vi "IO Test.vi"() -> ()   [LabVIEW 2009]
doc: "This example shows how to use Simulation Module and Control Design Toolkit together and how to transfer the controller from Design to Simulation. It also uses the 3D Picture Control Toolkit to animate the system.\nThis example is derived from the Quanser (www.quanser.com) 3 DOF Helicopter academic experiment."
uses:
  <vilib>/Simulation/Scripting/Companion Diagram/SimConfigNode/SimDog.xnode
  <vilib>/Simulation/Utility/SIMX Halt/SIMX Halt.xnode
  <vilib>/Simulation/Implementation/Shared/SIMSCR Execution Mode.ctl
  <vilib>/Simulation/Scripting/Companion Diagram/SimConfigNode/_simSolvers.ctl
  <vilib>/Simulation/Scripting/Companion Diagram/SimConfigNode/SimParams.ctl
  <vilib>/Simulation/Utility/Implementation/SIM Halt.vi
  NiRioSrv.dll
  <vilib>/Utility/error.llb/Error Cluster From Error Code.vi
  <vilib>/rvi/errors/niLvFpgaWhatHappensToTopLevelVI.ctl
  <vilib>/rvi/interface/common/niFpgaNodeNameForErrorReporting.ctl
  <vilib>/rvi/errors/niLvFpgaAdjustHostInterfaceError.vi
  <vilib>/rvi/interface/nirviReadWriteControl/nirviReadWriteControl.xnode
  FPGA Bitfiles/sbRIOController.lv~4B_sbRIO-9631_FPGA Main.vi.lvbitx
  <vilib>/userDefined/High Color/nirio_resource_hc.ctl
  <vilib>/rvi/interface/nirviOpenFPGA/nirviOpenFPGA.xnode
  RT/Set to PWM.vi
  <vilib>/rvi/interface/nirviCloseFPGA/nirviCloseFPGA.xnode
  FPGA/FPGA Main.vi
  RT/Read Encoder Data.vi
  <vilib>/Simulation/Implementation/Shared/SIM Bundle Sim Info.vi
  <vilib>/Simulation/Implementation/Shared/SIM Unbundle Sim Info.vi
  <vilib>/Platform/TimedLoop/XDataNode/wakeup.ctl
  <vilib>/Platform/TimedLoop/XDataNode/XDNodeRunTimeDep.lvlib
  <vilib>/Platform/TimedLoop/XDataNode/nitl_modes.ctl
  <vilib>/Platform/TimedLoop/XDataNode/timing_clust.ctl
  <vilib>/Platform/TimedLoop/XDataNode/XDataNode.xnode
  <vilib>/Simulation/Implementation/Shared/NILVSim_Initialize.vi
  <vilib>/Simulation/Implementation/Shared/NILVSim_FinishedLate.vi
  <vilib>/Simulation/Implementation/Shared/NILVSim_Manager.vi
  <vilib>/Simulation/Implementation/Shared/NILVSim_FinalizeModel.vi
  <vilib>/Simulation/Implementation/Shared/NILVSim_GetModelError.vi
  <vilib>/Platform/TimedLoop/XDataNode/loadlvalarms.vi
  <vilib>/Simulation/Implementation/Shared/SIM Fire Discrete SubVI.vi
  <vilib>/Simulation/Scripting/Editor Utilities/SIM subVI execution type.ctl
  <vilib>/Simulation/Scripting/Editor Utilities/SIM subVI tag data.ctl
  <vilib>/FPGAPlugInAG/sbRIO-9631/nirviIntfOpen_sbRIO-9631.vi
  FPGA/FPGA Main NoStartEnc.vi
  FPGA Bitfiles/sbRIOController.lv~4B_sbRIO-9631_FPGA Main NoStartE~C3.lvbitx
  <vilib>/FPGAPlugInAG/sbRIO-9631/nirviIntfClose_sbRIO-9631.vi
panel:
  in  "Fan Power (-1 to 1) 2":dbl(slide) scale=-1.0..1.0
  out "Trav Vel":dbl
  out "Pitch Vel":dbl
  out "Elv Vel":dbl
  in  "Fan Power (-1 to 1)":dbl(slide) scale=-1.0..1.0
  in  "stop":bool
  out "error out":errorcluster
  in  "GO":bool
  in  "Clock Divider (ticks)":u16=1
  in  "PWM Period (ticks)":u32=100000
  out "Measured Pitch Angle":dbl=0.00018032364824244914
  out "Measure Trav":dbl=14.22166948358761
  out "Measured Elevation":dbl=14.497088945408226
  # "X"
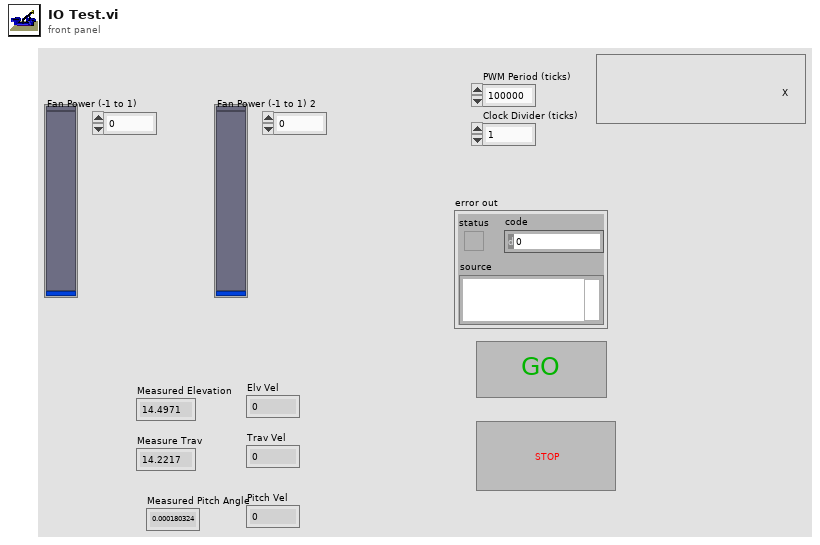
[diagram p1: front panel]
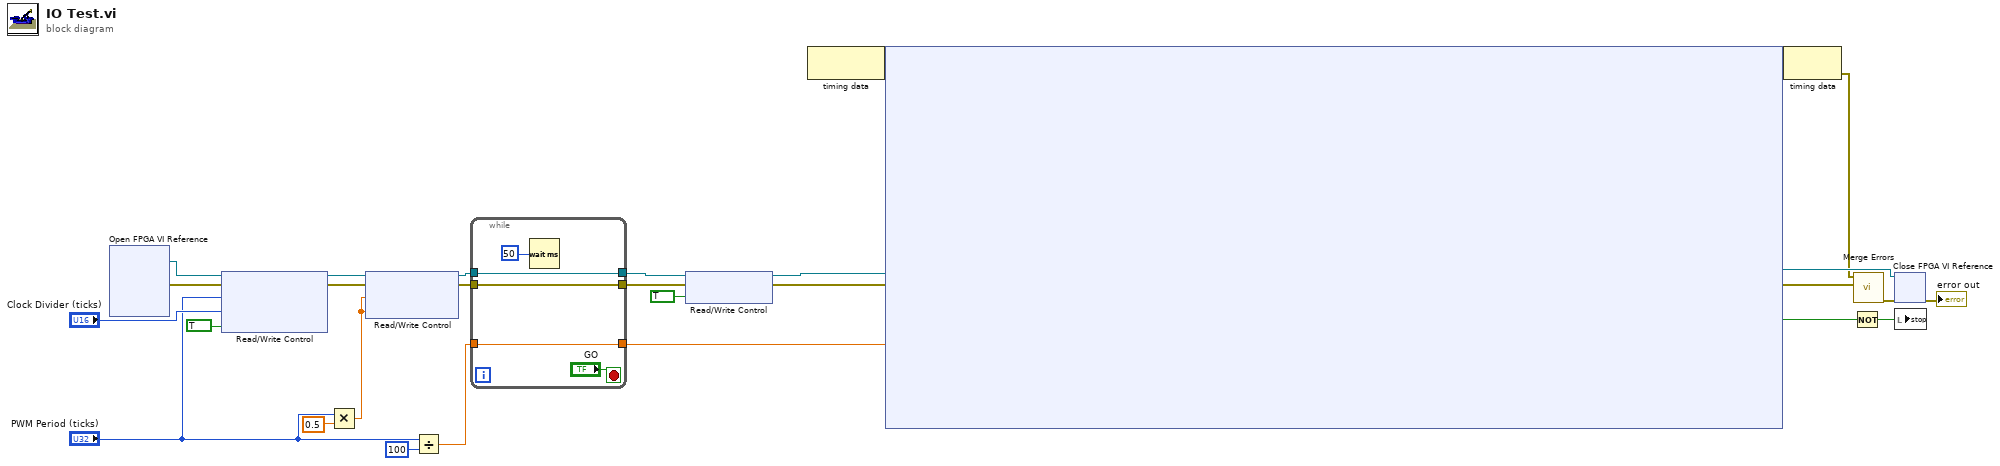
[diagram p0: block diagram]
diagram:
  n1 = xnode "Open FPGA VI Reference"() -> ("FPGA VI Reference Out"=w23:refnum<k20>, "error out"=w24:errorcluster)  [unwired: 2 in]
  n2 = xnode "Read/Write Control"("FPGA VI Reference In"=w23, "error in"=w24, "PWM Period (ticks)"="PWM Period (ticks)", "Clock Divider"="Clock Divider (ticks)", "ENC In Clock"=TRUE) -> ("FPGA VI Reference Out"=w8:refnum<k20>, "error out"=w9:errorcluster)
  n3 = Multiply(x="PWM Period (ticks)", y=sgl 0.5) -> (x*y=w12:sgl)
  n4 = xnode "Read/Write Control"("FPGA VI Reference In"=w8, "error in"=w9, "Fan High Time 1"=w12, "Fan High Time 2"=w12) -> ("FPGA VI Reference Out"=w6:refnum<k20>, "error out"=w7:errorcluster)
  n5 = Divide(x="PWM Period (ticks)", y=u32 100) -> (x/y=w21:dbl)
  n6 = while {
    tunnel: [w33] -> w20
    tunnel: w21 -> [w33]
    tunnel: w7 -> [w30]
    tunnel: w6 -> [w29]
    tunnel: [w30] -> w5
    tunnel: [w29] -> w4
    stop <- "GO" stop-if-true
    n7 = Wait (ms)(milliseconds to wait=u32 50) -> ()  [unwired: 1 out]
  }
  n8 = xnode "Read/Write Control"("FPGA VI Reference In"=w4, "error in"=w5, "Start Encoders"=TRUE) -> ("FPGA VI Reference Out"=w1:refnum<k20>, "error out"=w2:errorcluster)
  n9 = node-c288() -> (w28:variant)  [unwired: 1 in]
  n10 = node-c254 ("Simulation Loop")(w28, w2, w1, w20) -> (w27:variant, w16:errorcluster, w19:refnum<k20>, w11:bool)
  n11 = node-c288(w27) -> (w17:errorcluster)
  n12 = Not(x=w11) -> (.not. x?=w10:bool)
  n13 = call <vilib>:"Merge Errors.vi"("error in 2 (no error)"=w16, "error in 1 (no error)"=w17) -> ("error out"=w15:errorcluster)  [unwired: 5 in]
  n14 = xnode "Close FPGA VI Reference"("FPGA VI Reference In"=w19, "error in"=w15) -> ("error out"=→"error out":errorcluster)
  n15 = local write "stop"(w10) -> ()
